vi "_CallShell.vi"() -> ()   [LabVIEW 2019, in "lv-providershell-example2.lvlib"]
uses:
  lv-providershell-example2.lvlib
  src/VIProviderShellHelper.lvclass
panel:
  out "Cluster 2":T1
  in  "stop":bool
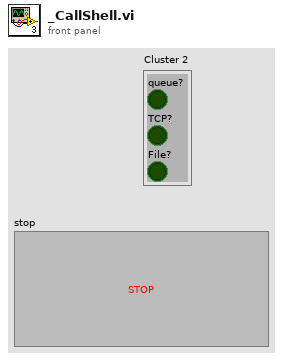
[diagram p1: front panel]
types:
  T1 = cluster{"queue?":bool, "TCP?":bool, "File?":bool}
  T2 = cluster{"queue":refnum<queue>, "TCP":refnum<k5>, "File":refnum<file>}
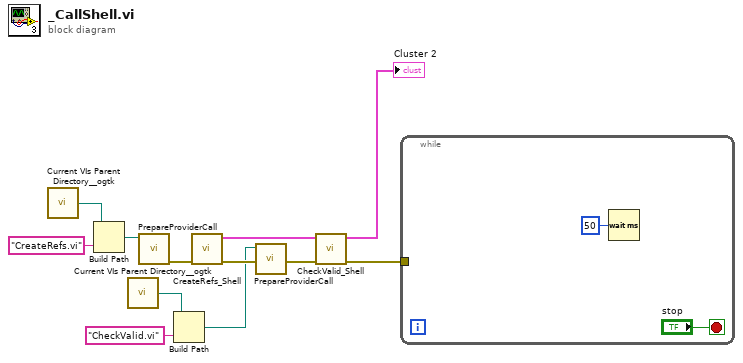
[diagram p0: block diagram]
diagram:
  n1 = call <userlib>:"Current VIs Parent Directory__ogtk.vi"() -> ("Parent Directory (+ Relative)"=w8:path)  [unwired: 5 in]
  n2 = Build Path(base path=w8, name or relative path="CreateRefs.vi") -> (appended path=w7:path)
  n3 = call <userlib>:"Current VIs Parent Directory__ogtk.vi"() -> ("Parent Directory (+ Relative)"=w4:path)  [unwired: 5 in]
  n4 = call "PrepareProviderCall.vi"("ProviderCotentVI Path"=w7) -> ("error out"=w11:errorcluster)  [unwired: 10 in]
  n5 = Build Path(base path=w4, name or relative path="CheckValid.vi") -> (appended path=w3:path)
  n6 = call "CreateRefs_Shell.vi"("error in (no error)"=w11) -> ("error out"=w9:errorcluster, "Cluster"=w12:T2)  [unwired: 9 in]
  n7 = call "PrepareProviderCall.vi"("error in (no error)"=w9, "ProviderCotentVI Path"=w3) -> ("error out"=w10:errorcluster)  [unwired: 9 in]
  n8 = call "CheckValid_Shell.vi"("error in (no error)"=w10, "Cluster"=w12) -> ("error out"=w2:errorcluster, "Cluster 2"=→"Cluster 2":T1)  [unwired: 8 in]
  n9 = while {
    tunnel: w2 -> [_]
    stop <- "stop" stop-if-true
    n10 = Wait (ms)(milliseconds to wait=u32 50) -> ()  [unwired: 1 out]
  }
